vi "SendData.vi"(8 "error in (no error)":errorcluster, 11 "Communication in":refnum<class "Communication.lvclass">) -> (0 "error out":errorcluster, 2 "Data out":refnum<class "Data.lvclass">, 3 "Communication out":refnum<class "Communication.lvclass">)   [LabVIEW 2023, in "Communication.lvclass"]
uses:
  Communication.lvclass
  Data/Data.lvclass
  Communication.lvclass/Communication.ctl
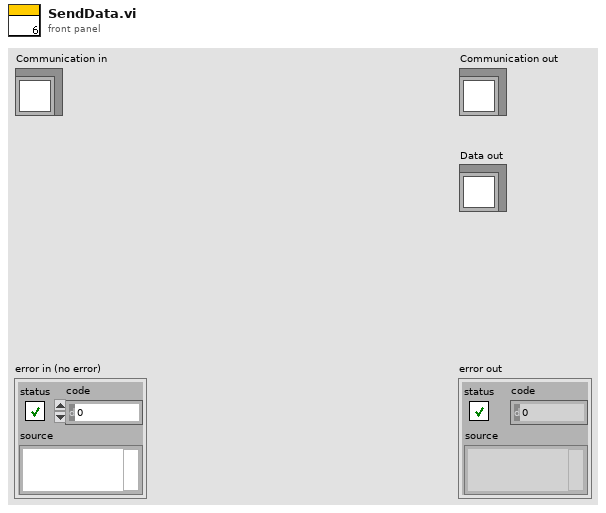
[diagram p1: front panel]
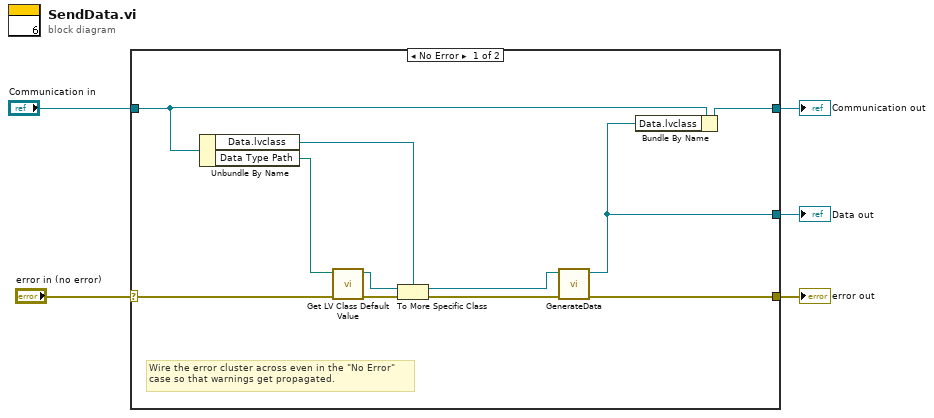
[diagram p0: block diagram]
diagram:
  n1 = case shown="No Error" "error in (no error)" {
    selector: "error in (no error)" -> [w16 w18]
    tunnel: [w15 w18] -> w4
    tunnel: [w13 w17] -> w2
    tunnel: "Communication in" -> [w14 w17]
    tunnel: [w12 _] -> w1
    frame No Error {
      # "Wire the error cluster across even in the \"No Error\"\ncase so that warnings get propagated."
      n2 = Unbundle By Name(w14) -> ("Data.lvclass"=w7:refnum<class "Data.lvclass">, "Data Type Path"=w10:path)
      n3 = call <vilib>:"Get LV Class Default Value.vi"("error in (no error)"=w16, "class path"=w10) -> ("error out"=w11:errorcluster, "object"=w8:refnum<class>)  [unwired: 8 in]
      n4 = To More Specific Class(target class=w7, reference=w8, error in=w11) -> (specific class reference=w6:refnum<class "Data.lvclass">, error out=w9:errorcluster)
      n5 = call-dynamic "GenerateData.vi"("error in (no error)"=w9, "Data in"=w6) -> ("error out"=w15:errorcluster, "Data out"=w12:refnum<class "Data.lvclass">)  [unwired: 8 in]
      n6 = Bundle By Name(cluster=w14, "Data.lvclass"=w12) -> (w13:refnum<class "Communication.lvclass">)
    }
    frame Error {
    }
  }
  "error out" <- w4
  "Communication out" <- w2
  "Data out" <- w1
